vi "GET_Decision_about_TTL_2.vi"(8 "Error In":errorcluster, 10 "Settings cluster":T12={"Defaults"={"Default User"=0.0, "VISA Resource Name "="", "Histogram parameters"={"max"=0.0, "min"=0.0, "# bins"=0, "threshold"=0.0, "thr. type"=enum."higher accepted"}}, "Recording and saving"={"Researcher name"="", "Name prefix"="", "Data post-processing"={"Filter type"=enum."None", "Length"=0, "Order"=0}, "Stop at"=0.0, "\"Stop at\" enabled"=FALSE, "Default save folder path"=path "", "Acquisition FPS"=enum."Max"}, "Geometry"={"Sensor board size"=enum."", "Bridge swap"=FALSE, "Twisted neck"=FALSE, "Bridge H. offset"=0.0, "Bridge V. offset"=0.0, "Magnets orientation"=0.0, "Cage type"=0, "Cage parameters"={"Round"=variant(i16 0), "Square"=variant(u16 0), "Donut-maze"=variant(u16 0), "T-maze"=variant(u8 0), "Sociability-maze"=variant(u8 0)}}, "IO parameters"={"IO general config."=0, "IO 1 configuration"=0, "IO 2 configuration"=0, "IO 3 configuration"=0, "IO 4 configuration"=0, "Activate ext. RS-232"=0, "IO inversion config."=0, "Sync capability"=0}, "Conditions presets array"=[], "Calibration parameters"={"Timing calibration sw/hw"=0.0, "True FPS"=0.0, "True frame time, s"=0.0, "Disp. calibration info"=[]}, "Settings loaded OK"=FALSE} {"Calibration parameters"."True frame time, s" format="%.10g"; "Calibration parameters"."Disp. calibration info"."Speed, µl per ms" format="%.3g"; "Calibration parameters"."True FPS" format="%.10g"; "Calibration parameters"."Timing calibration sw/hw" format="%.10g"; "Conditions presets array"."Specifier(s)"."Validity criteria(s)"."Validity value" min=0.0 step=0.1 format="%.2g"; "Conditions presets array"."Specifier(s)"."Value" step=1.0 format="%#.2g"; "Recording and saving"."Data post-processing"."Order" min=3 max=11 step=2; "Recording and saving"."Data post-processing"."Length" min=5 max=301 step=2; "Geometry"."Cage type" items=["Round", "Square", "Donut-maze", "T-maze", "Sociability maze", ""]}, 11 "Current animal coordinates and stats":T9 {"Measurements and statistics"."Running, perc. of time" format="%05.2f"}) -> (0 "Error Out":errorcluster, 3 "To be activated":bool[](array[boolean]))   [LabVIEW 2018, in "Tracker.lvlib"]
uses:
  Tracker.lvlib
  Controls/CTL_Settings_cluster.ctl
  Controls/CTL_Histogram_parameters.ctl
  Controls/CTL_Filter_selector.ctl
  Controls/CTL_Acquisition_speed_selector.ctl
  Common/Typedefs/CTL_Segmented_plot_parameters_2.ctl
  Libraries/Cage Diagram/Typedefs/CTL_Cage_type.ctl
  Controls/CTL_Cage_all_segmentation_params_set.ctl
  Controls/CTL_IO_params_cluster.ctl
  Controls/CTL_Conditions_Array.ctl
  Controls/CTL_Conditions_Cluster.ctl
  Controls/CTL_Condition_type.ctl
  Controls/CTL_Comparison_type.ctl
  Controls/CTL_Validity_check_criteria.ctl
  Controls/CTL_Response_info.ctl
  Controls/CTL_Condition_response_type.ctl
  Controls/CTL_Reponse_port_info.ctl
  Controls/CTL_Calibration_parameters.ctl
  Controls/CTL_Dispenser_calibration_info.ctl
  Controls/CTL_Full_data_frame.ctl
  Controls/CTL_Animal_Coordinates_and_Speed.ctl
  Controls/CTL_Measurements_and_Statistics.ctl
  <vilib>/ptbypt/NI_PtbyPt.lvlib
  Common_Resources.lvlib
  Libraries/Cage Diagram/Cage Diagram.lvlib
panel:
  out "Conditions presets array":T1 {"Specifier(s)"."Validity criteria(s)"."Validity value" min=0.0 step=0.1 format="%.2g"; "Specifier(s)"."Value" step=1.0 format="%#.2g"}
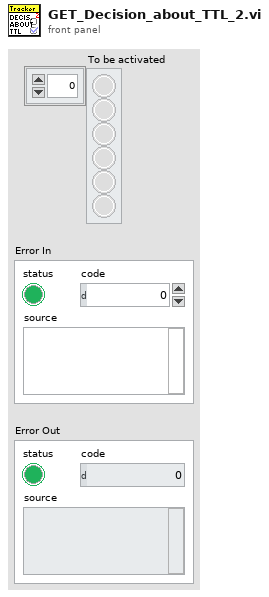
[diagram p1: front panel]
types:
  T1 = typedef "Common_Resources.lvlib/CTL_Conditions_Array.ctl" = T2[]
  T2 = typedef "Common_Resources.lvlib/CTL_Conditions_Cluster.ctl" = cluster{"Enabled":bool, "Name":string, "Specifier(s)":cluster{"Specifier enabled":bool, "Condition type":T3, "Comparison type":T4, "Value":dbl, "Validity criteria(s)":cluster{"V. check enabled":bool, "Criteria":T5, "Validity value":dbl}[]}[], "Response":T6, "Has been set":bool}
  T3 = typedef "Common_Resources.lvlib/CTL_Condition_type.ctl" = enum16{"Speed", "Zone", "Angle to wall"}
  T4 = typedef "Common_Resources.lvlib/CTL_Comparison_type.ctl" = enum16{"Less", "Less or Equal", "Equal", "Greater or Equal", "Greater", "Not Equal"}
  T5 = typedef "Common_Resources.lvlib/CTL_Validity_check_criteria.ctl" = enum16{"Running bout (seconds)", "Running bout (meters)"}
  T6 = typedef "Common_Resources.lvlib/CTL_Response_info.ctl" = cluster{"Response type":T7, "TTL port":T8, "TTL pulse length, ms":dbl}
  T7 = typedef "Common_Resources.lvlib/CTL_Condition_response_type.ctl" = enum16{"None", "Air puff", "Liquid reward", "TTL pulse", "TTL pulse (ubr)", "TTL signal"}
  T8 = typedef "Common_Resources.lvlib/CTL_Reponse_port_info.ctl" = enum16{"Port 1", "Port 2", "Port 3", "Port 4"}
  T9 = typedef "Common_Resources.lvlib/CTL_Full_data_frame.ctl" = cluster{"Times":cluster{"ms since ON":u32, "delta time":u32, "Frame timestamp":timestamp}, "TTLs":cluster{"TTL input":i16, "TTL output":i16}, "Animal coordinates":T10, "Magnets coords raw":cluster{"X1 raw":dbl, "Y1 raw":dbl, "X2 raw":dbl, "Y2 raw":dbl}, "Measurements and statistics":T11}
  T10 = typedef "Common_Resources.lvlib/CTL_Animal_Coordinates_and_Speed.ctl" = cluster{"R from center":dbl, "phi (mouse angular position in the cage)":dbl, "alpha (mouse rot. angle)":dbl, "X":dbl, "Y":dbl, "theta (from center towards mouse)":dbl, "beta (cage rot. against mouse)":dbl, "w (mouse angle to wall)":dbl, "Speed (filtered)":dbl}
  T11 = typedef "Common_Resources.lvlib/CTL_Measurements_and_Statistics.ctl" = cluster{"Zone #":i8, "Histogram":dbl[], "Running, perc. of time":dbl, "Run, meters":dbl, "Avg. speed":dbl}
  T12 = typedef "Common_Resources.lvlib/CTL_Settings_cluster.ctl" = cluster{"Defaults":cluster{"Default User":dbl, "VISA Resource Name ":string, "Histogram parameters":T13}, "Recording and saving":cluster{"Researcher name":string, "Name prefix":string, "Data post-processing":T14, "Stop at":dbl, "\"Stop at\" enabled":bool, "Default save folder path":path, "Acquisition FPS":T15}, "Geometry":T16, "IO parameters":T19, "Conditions presets array":T1, "Calibration parameters":T20, "Settings loaded OK":bool}
  T13 = typedef "Common_Resources.lvlib/CTL_Histogram_parameters.ctl" = cluster{"max":dbl, "min":dbl, "# bins":i32, "threshold":dbl, "thr. type":enum16{"higher accepted", "lower accepted"}}
  T14 = typedef "Common_Resources.lvlib/CTL_Filter_selector.ctl" = cluster{"Filter type":enum16{"None", "Savitzky-Golay"}, "Length":i32, "Order":i32}
  T15 = typedef "Common_Resources.lvlib/CTL_Acquisition_speed_selector.ctl" = enum16{"Max", "Optimal", "Eco"}
  T16 = typedef "Common_Resources.lvlib/CTL_Segmented_plot_parameters_2.ctl" = cluster{"Sensor board size":enum16{"", "Large"}, "Bridge swap":bool, "Twisted neck":bool, "Bridge H. offset":sgl, "Bridge V. offset":sgl, "Magnets orientation":sgl, "Cage type":T17, "Cage parameters":T18}
  T17 = typedef "Cage Diagram.lvlib/CTL_Cage_type.ctl" = u16
  T18 = typedef "Common_Resources.lvlib/CTL_Cage_all_segmentation_params_set.ctl" = cluster{"Round":variant, "Square":variant, "Donut-maze":variant, "T-maze":variant, "Sociability-maze":variant}
  T19 = typedef "Common_Resources.lvlib/CTL_IO_params_cluster.ctl" = cluster{"IO general config.":u16, "IO 1 configuration":u16, "IO 2 configuration":u16, "IO 3 configuration":u16, "IO 4 configuration":u16, "Activate ext. RS-232":u16, "IO inversion config.":u16, "Sync capability":u8}
  T20 = typedef "Common_Resources.lvlib/CTL_Calibration_parameters.ctl" = cluster{"Timing calibration sw/hw":dbl, "True FPS":dbl, "True frame time, s":dbl, "Disp. calibration info":T21}
  T21 = typedef "Common_Resources.lvlib/CTL_Dispenser_calibration_info.ctl" = cluster{"Channel":u8, "Speed, µl per ms":dbl}[]
  T22 = cluster{"Specifier enabled":bool, "Condition type":T3, "Comparison type":T4, "Value":dbl, "Validity criteria(s)":cluster{"V. check enabled":bool, "Criteria":T5, "Validity value":dbl}[]}[]
  T23 = cluster{"V. check enabled":bool, "Criteria":T5, "Validity value":dbl}[]
  T24 = cluster{"V. check enabled":bool, "Criteria":T5, "Validity value":dbl}
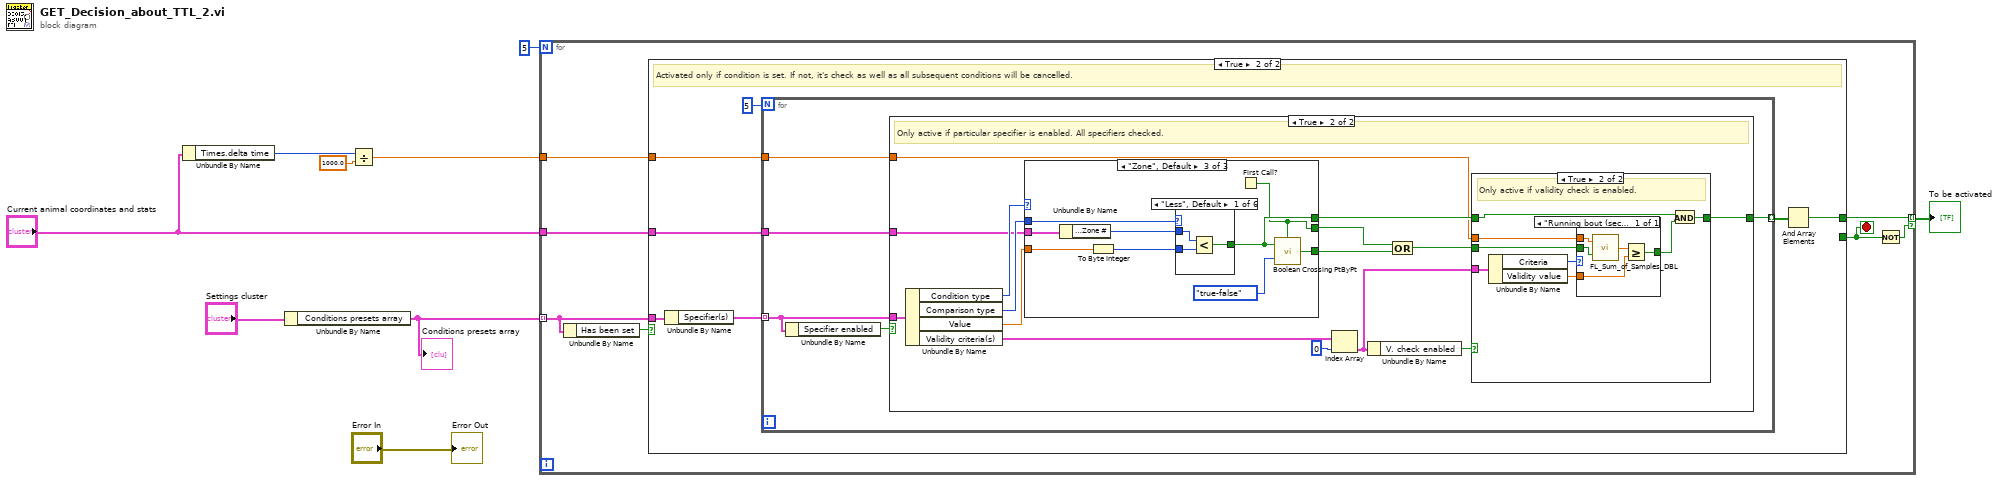
[diagram p0: block diagram]
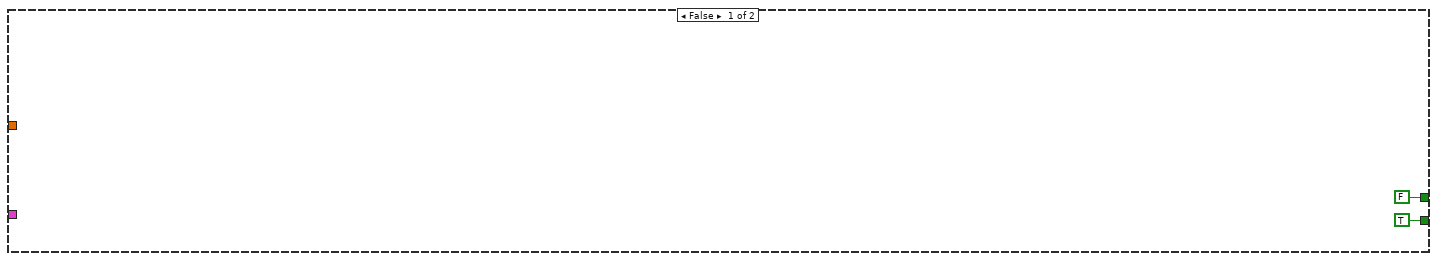
[diagram p2: hidden frame]
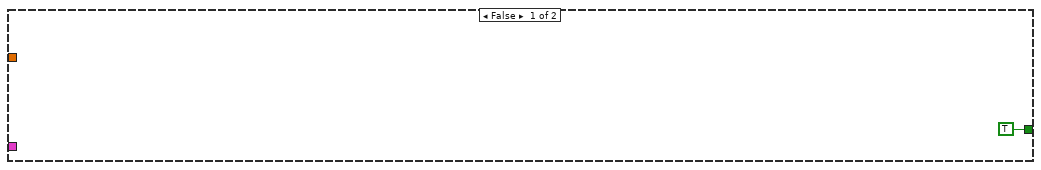
[diagram p3: hidden frame]
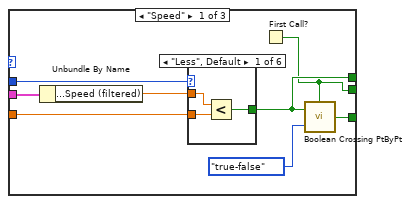
[diagram p4: hidden frame]
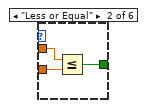
[diagram p5: hidden frame]
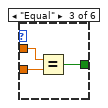
[diagram p6: hidden frame]
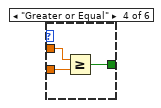
[diagram p7: hidden frame]
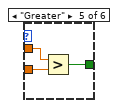
[diagram p8: hidden frame]
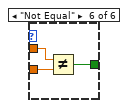
[diagram p9: hidden frame]
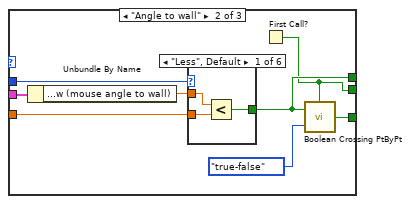
[diagram p10: hidden frame]
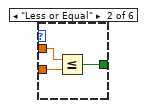
[diagram p11: hidden frame]
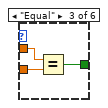
[diagram p12: hidden frame]
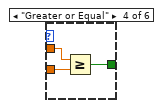
[diagram p13: hidden frame]
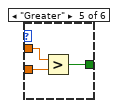
[diagram p14: hidden frame]
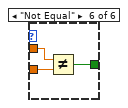
[diagram p15: hidden frame]
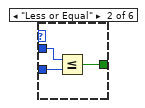
[diagram p16: hidden frame]
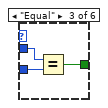
[diagram p17: hidden frame]
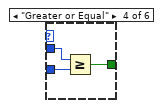
[diagram p18: hidden frame]
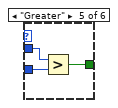
[diagram p19: hidden frame]
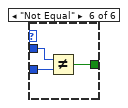
[diagram p20: hidden frame]
diagram:
  n1 = Unbundle By Name("Current animal coordinates and stats") -> ("Times.delta time"=w4:u32)
  n2 = Unbundle By Name("Settings cluster") -> ("Conditions presets array"=w8:T1)
  "Conditions presets array" <- w8
  n3 = Divide(x=w4, y=1000.0) -> (x/y=w2:dbl)
  n4 = for {
    N: 5 -> [_]
    tunnel: w8 -> [w16] mode=indexing
    tunnel: [w14] -> w6 mode=indexing if=w10
    tunnel: "Current animal coordinates and stats" -> [w13]
    tunnel: w2 -> [w12]
    stop <- w11 stop-if-true
    n5 = Unbundle By Name(w16) -> ("Has been set"=w15:bool)
    n6 = case shown="True" w15 {
      tunnel: w16 -> [_ w25]
      tunnel: [TRUE _] -> w11
      tunnel: [FALSE w21] -> w14
      tunnel: w13 -> [_ w20]
      tunnel: w12 -> [_ w19]
      frame False {
      }
      frame True {
        # "Activated only if condition is set. If not, it's check as well as all subsequent conditions will be cancelled."
        n7 = Unbundle By Name(w25) -> ("Specifier(s)"=w23:T22)
        n8 = for {
          N: 5 -> [_]
          tunnel: w23 -> [w29] mode=indexing
          tunnel: [w28] -> w22 mode=indexing
          tunnel: w20 -> [w27]
          tunnel: w19 -> [w26]
          n9 = Unbundle By Name(w29) -> ("Specifier enabled"=w30:bool)
          n10 = case shown="True" w30 {
            tunnel: w29 -> [_ w46]
            tunnel: [TRUE w35] -> w28
            tunnel: w27 -> [_ w38]
            tunnel: w26 -> [_ w36]
            frame False {
            }
            frame True {
              # "Only active if particular specifier is enabled. All specifiers checked."
              n11 = Unbundle By Name(w46) -> ("Condition type"=w43:T3, "Comparison type"=w40:T4, "Value"=w41:dbl, "Validity criteria(s)"=w45:T23)
              n12 = case shown="\"Zone\", Default" w43 {
                tunnel: w38 -> [w54 w80 w107]
                tunnel: w41 -> [w52 w78 w105]
                tunnel: w40 -> [w51 w77 w104]
                tunnel: [w50 w76 w101] -> w37
                tunnel: [w49 w75 w100] -> w33
                tunnel: [w47 w73 w99] -> w32
                frame "Speed" {
                  n13 = Unbundle By Name(w54) -> ("Animal coordinates.Speed (filtered)"=w53:dbl)
                  n14 = case shown="\"Less\", Default" w51 {
                    tunnel: w53 -> [w57 w60 w63 w66 w69 w72]
                    tunnel: [w56 w59 w62 w65 w68 w71] -> w50
                    tunnel: w52 -> [w55 w58 w61 w64 w67 w70]
                    frame "Less", Default {
                      n15 = Less?(x=w57, y=w55) -> (x < y?=w56:bool)
                    }
                    frame "Less or Equal" {
                      n16 = Less Or Equal?(x=w60, y=w58) -> (x <= y?=w59:bool)
                    }
                    frame "Equal" {
                      n17 = Equal?(x=w63, y=w61) -> (x = y?=w62:bool)
                    }
                    frame "Greater or Equal" {
                      n18 = Greater Or Equal?(x=w66, y=w64) -> (x >= y?=w65:bool)
                    }
                    frame "Greater" {
                      n19 = Greater?(x=w69, y=w67) -> (0:w68:bool)
                    }
                    frame "Not Equal" {
                      n20 = Not Equal?(x=w72, y=w70) -> (x != y?=w71:bool)
                    }
                  }
                  n21 = First Call?() -> (First Call?: T/F=w47:bool)
                  n22 = call <vilib>:"Boolean Crossing PtByPt.vi"("initialize"=w47, "direction"=enum16{"either", "false-true", "true-false"}."true-false", "input"=w50) -> ("crossing"=w49:bool)
                }
                frame "Angle to wall" {
                  n23 = Unbundle By Name(w80) -> ("Animal coordinates.w (mouse angle to wall)"=w79:dbl)
                  n24 = case shown="\"Less\", Default" w77 {
                    tunnel: w79 -> [w83 w86 w89 w92 w95 w98]
                    tunnel: [w82 w85 w88 w91 w94 w97] -> w76
                    tunnel: w78 -> [w81 w84 w87 w90 w93 w96]
                    frame "Less", Default {
                      n25 = Less?(x=w83, y=w81) -> (x < y?=w82:bool)
                    }
                    frame "Less or Equal" {
                      n26 = Less Or Equal?(x=w86, y=w84) -> (x <= y?=w85:bool)
                    }
                    frame "Equal" {
                      n27 = Equal?(x=w89, y=w87) -> (x = y?=w88:bool)
                    }
                    frame "Greater or Equal" {
                      n28 = Greater Or Equal?(x=w92, y=w90) -> (x >= y?=w91:bool)
                    }
                    frame "Greater" {
                      n29 = Greater?(x=w95, y=w93) -> (0:w94:bool)
                    }
                    frame "Not Equal" {
                      n30 = Not Equal?(x=w98, y=w96) -> (x != y?=w97:bool)
                    }
                  }
                  n31 = First Call?() -> (First Call?: T/F=w73:bool)
                  n32 = call <vilib>:"Boolean Crossing PtByPt.vi"("initialize"=w73, "direction"=enum16{"either", "false-true", "true-false"}."true-false", "input"=w76) -> ("crossing"=w75:bool)
                }
                frame "Zone", Default {
                  n33 = Unbundle By Name(w107) -> ("Measurements and statistics.Zone #"=w106:i8)
                  n34 = To Byte Integer(number=w105) -> (8bit integer=w103:i8)
                  n35 = case shown="\"Less\", Default" w104 {
                    tunnel: w106 -> [w110 w113 w116 w119 w122 w125]
                    tunnel: [w109 w112 w115 w118 w121 w124] -> w101
                    tunnel: w103 -> [w108 w111 w114 w117 w120 w123]
                    frame "Less", Default {
                      n36 = Less?(x=w110, y=w108) -> (x < y?=w109:bool)
                    }
                    frame "Less or Equal" {
                      n37 = Less Or Equal?(x=w113, y=w111) -> (x <= y?=w112:bool)
                    }
                    frame "Equal" {
                      n38 = Equal?(x=w116, y=w114) -> (x = y?=w115:bool)
                    }
                    frame "Greater or Equal" {
                      n39 = Greater Or Equal?(x=w119, y=w117) -> (x >= y?=w118:bool)
                    }
                    frame "Greater" {
                      n40 = Greater?(x=w122, y=w120) -> (0:w121:bool)
                    }
                    frame "Not Equal" {
                      n41 = Not Equal?(x=w125, y=w123) -> (x != y?=w124:bool)
                    }
                  }
                  n42 = First Call?() -> (First Call?: T/F=w99:bool)
                  n43 = call <vilib>:"Boolean Crossing PtByPt.vi"("initialize"=w99, "direction"=enum16{"either", "false-true", "true-false"}."true-false", "input"=w101) -> ("crossing"=w100:bool)
                }
              }
              n44 = Index Array(array=w45, index=0) -> (element=w39:T24)
              n45 = Unbundle By Name(w39) -> ("V. check enabled"=w42:bool)
              n46 = Compound Arithmetic op=OR(w32, w33) -> (w34:bool)
              n47 = case shown="True" w42 {
                tunnel: w37 -> [w126 w130]
                tunnel: [w126 w131] -> w35
                tunnel: w39 -> [_ w134]
                tunnel: w36 -> [_ w128]
                tunnel: w34 -> [_ w127]
                frame False {
                }
                frame True {
                  # "Only active if validity check is enabled."
                  n48 = Unbundle By Name(w134) -> ("Criteria"=w133:T5, "Validity value"=w132:dbl)
                  n49 = case shown="\"Running bout (seconds)\", Default" w133 {
                    tunnel: w132 -> [w139]
                    tunnel: w127 -> [w135]
                    tunnel: [w138] -> w129
                    tunnel: w128 -> [w137]
                    frame "Running bout (seconds)", Default {
                      n50 = call "FL_Sum_of_Samples_DBL.vi"("Reset?"=w135, "Input sample"=w137) -> ("Sum of samples"=w136:dbl)
                      n51 = Greater Or Equal?(x=w136, y=w139) -> (x >= y?=w138:bool)
                    }
                  }
                  n52 = And(x=w130, y=w129) -> (x .and. y?=w131:bool)
                }
              }
            }
          }
        }
        n53 = And Array Elements(Boolean array=w22) -> (logical AND=w21:bool)
      }
    }
    n54 = Not(x=w11) -> (.not. x?=w10:bool)
  }
  "To be activated" <- w6
  "Error Out" <- "Error In"
